vi "serialWrite_p.vi"(2 "string to write":string, 3 "serialBoard":u16(ring) items=["DEVIL", "M17"], 4 "timeOut [ms] (1000)":i32=1000, 5 "subID2 (0)":u32, 6 "subID1 (0)":u32 format="%.0x", 7 "baseAdderess":u32=3774873600 format="%.0x") -> (0 "errorSpec":i32, 1 "errorCode":cdb format="%.2f")   [LabVIEW 2010]
doc: "writes the content of the output buffer of the serial port specified by \"subID1\" and \"subID2\".\nWARNING: remember to setup the serial channel before running this routine using:\n1. \"serialInitialize.vi\" for hardware setup;\n2. \"serialConfigure\" for software setup."
uses:
  <userlib>/libcommon_serial/libcommon_serial.lvlib
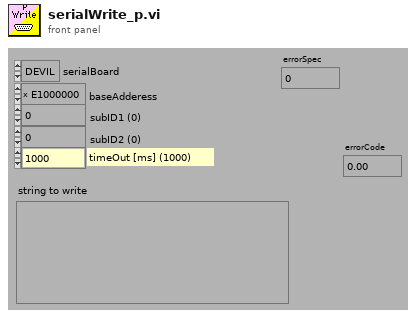
[diagram p1: front panel]
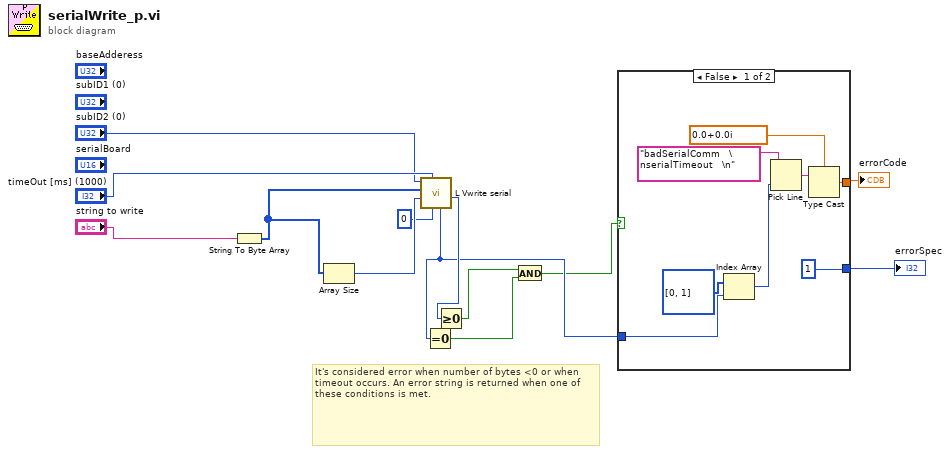
[diagram p0: block diagram]
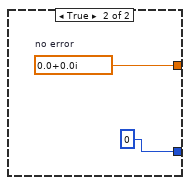
[diagram p2: hidden frame]
diagram:
  # "It's considered error when number of bytes <0 or when timeout occurs. An error string is returned when one of these conditions is met."
  n1 = String To Byte Array(string="string to write") -> (unsigned byte array=w10:u8[])
  n2 = Array Size(array=w10) -> (size(s)=w9:i32)
  n3 = call <userlib>:"L Vwrite serial.vi"("timoccur"=0, "timeo"="timeOut [ms] (1000)", "bsize"=w9, "buf"=w10, "resourceId"="subID2 (0)") -> ("byte written"=w4:i32, "timoccur out"=w3:i32)  [unwired: 3 in, 2 out]
  n4 = Equal To 0?(x=w3) -> (x = 0?=w6:bool)
  n5 = Greater Or Equal To 0?(x=w4) -> (x >= 0?=w5:bool)
  n6 = And(x=w5, y=w6) -> (x .and. y?=w2:bool)
  n7 = case shown="False" w2 {
    tunnel: [w18 w23] -> w7
    tunnel: w3 -> [w15 _]
    tunnel: [1 0] -> w1
    frame False {
      n8 = Index Array(array=i32[] [0, 1], index=w15) -> (element=w17:i32)
      n9 = Pick Line(multi-line string="badSerialComm   \nserialTimeout   \n", line index=w17) -> (output string=w20:string)  [unwired: 1 in]
      n10 = Type Cast(type=cdb 0.0+0.0i, x=w20) -> (*(type *) &x=w18:cdb)
    }
    frame True {
      w23 = cdb 0.0+0.0i  # no error
    }
  }
  "errorCode" <- w7
  "errorSpec" <- w1
